vi "Find Distance Between Points.vi"(1 "position 2":cluster{"x position":i16, "y position":i16}, 2 "position 1":cluster{"x position":i16, "y position":i16}) -> (0 "distance":dbl)   [LabVIEW 2010]
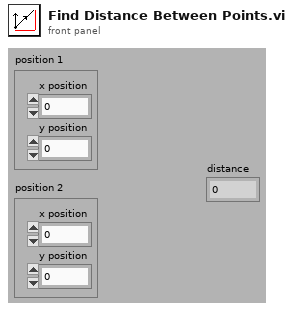
[diagram p1: front panel]
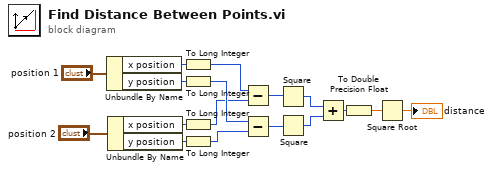
[diagram p0: block diagram]
diagram:
  n1 = Unbundle By Name("position 1") -> ("x position"=w6:i16, "y position"=w9:i16)
  n2 = Unbundle By Name("position 2") -> ("x position"=w7:i16, "y position"=w8:i16)
  n3 = To Long Integer(number=w6) -> (32bit integer=w4:i32)
  n4 = To Long Integer(number=w9) -> (32bit integer=w3:i32)
  n5 = To Long Integer(number=w7) -> (32bit integer=w2:i32)
  n6 = To Long Integer(number=w8) -> (32bit integer=w1:i32)
  n7 = Subtract(x=w4, y=w2) -> (x-y=w17:i32)
  n8 = Subtract(x=w3, y=w1) -> (x-y=w16:i32)
  n9 = Square(x=w17) -> (x^2=w14:i32)
  n10 = Square(x=w16) -> (x^2=w15:i32)
  n11 = Add(x=w14, y=w15) -> (x+y=w13:i32)
  n12 = To Double Precision Float(number=w13) -> (double precision float=w5:dbl)
  n13 = Square Root(x=w5) -> (sqrt(x)=→"distance":dbl)
